vi "GEN_True String to Bool.vi"(10 "string in":string) -> (2 "true?":bool)   [LabVIEW 2016]
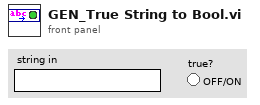
[diagram p1: front panel]
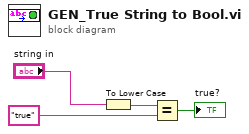
[diagram p0: block diagram]
diagram:
  n1 = To Lower Case(string="string in") -> (all lower case string=w4:string)
  n2 = Equal?(x=w4, y="true" ("string in")) -> (x = y?=→"true?":bool)
